vi "TAS-multiwavelength.vi"() -> ()   [LabVIEW 2012]
uses:
  <vilib>/DAQmx/read.llb/DAQmx Read (Analog DBL 1Chan 1Samp).vi
  <vilib>/DAQmx/miscellaneous.llb/DAQmx Fill In Error Info.vi
panel:
  out "Light Level":cluster{"X":dbl, "Y":dbl}[](graph)
  in  "ABORT LL SCAN":bool
  out "Monos moving":bool
  out "error out 2":errorcluster
  out "error out":errorcluster
  out "Detector Blaze":dbl
  out "Lamp Blaze":dbl
  out "Lamp WL":dbl
  out "Detector WL":dbl
  out "Laser Shutter State":string
  in  "START SCAN":bool
  out "Scanning":bool
  out "Osc. Time Range":string
  out "Laser State":string
  out "Total Steps":string
  out "Current Step":string
  out "Light Level (V)":dbl
  out "OPO Shutter State":string
  out "Total Averages":string
  out "Current Average":string
  out "Detector State":string
  out "Lamp State":string
  in  "SetTimeRange":bool
  in  "Time range":string(combo)
  in  "Averages per WL":dbl
  in  "Change Grating":bool
  in  "ScanLightLevel":bool
  in  "SAVE":bool
  in  "LASER OFF":bool
  in  "ABORT SCAN":bool
  in  "LASER ON":bool
  in  "Grating choice":dbl=1.0 min=1.0 max=2.0 step=1.0
  in  "Wavelength Range":string
  out "Scan Progress":u8(slide) scale=0.0..100.0
  in  "Exit":bool
  out "Transient Absorption":dbl[][](graph)
  # "Current state"
  # "WARNING: THIS PROGRAM IS UNDER\nDEVELOPMENT AND MUST NOT BE USED"
  # "Wavelength Settings"
  # "MATLAB notation. Leave a gap\nat the excitation WL. Example:\n\"300:1:450 500:1:700\" scans 300-450nm with a step of 1nm, leaves\na 50 nm gap around the excitation WL 475 nm, then continues scanning 500-700nm with a step of 1 nm."
  # "Maximum transmission occurs at\nblaze WL.\n\nBlaze 1 = 350 nm, Blaze 2 = 750 nm."
  # "Time range and averaging"
  # "Reserved For Future Convenience Functions"
  # "System"
  # "Light Level"
  # "Check if the light level is good over the\nselected wavelength range. Optimum 1.25 V, don't exceed 1.5 V at any WL."
  # "Remember to set the filter knobs manually according to table:"
  # "Time Range:          High Pass:          Low Pass:\n100 ns/div              10 us                   10 ns\n1 us/div                  100 us                 100 ns\n10 us/div                1 ms                    1 us\n100 us/div              10 ms                  10 us"
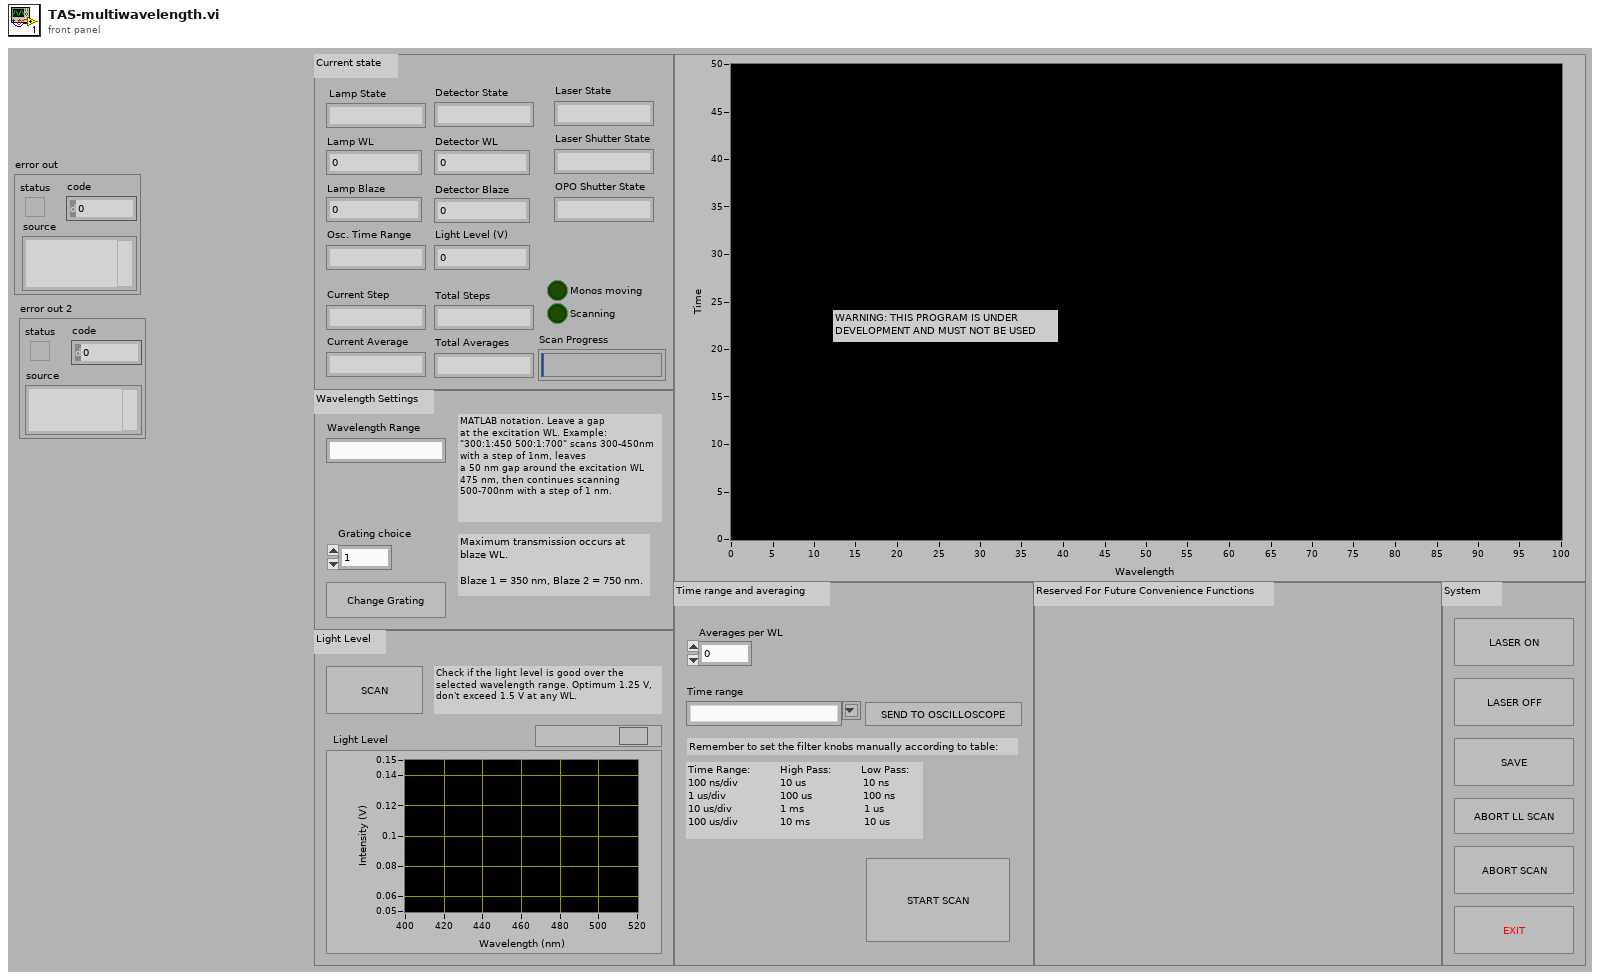
[diagram p1: front panel]
types:
  T1 = typedef "Cornerstone deviceID.ctl" = i32
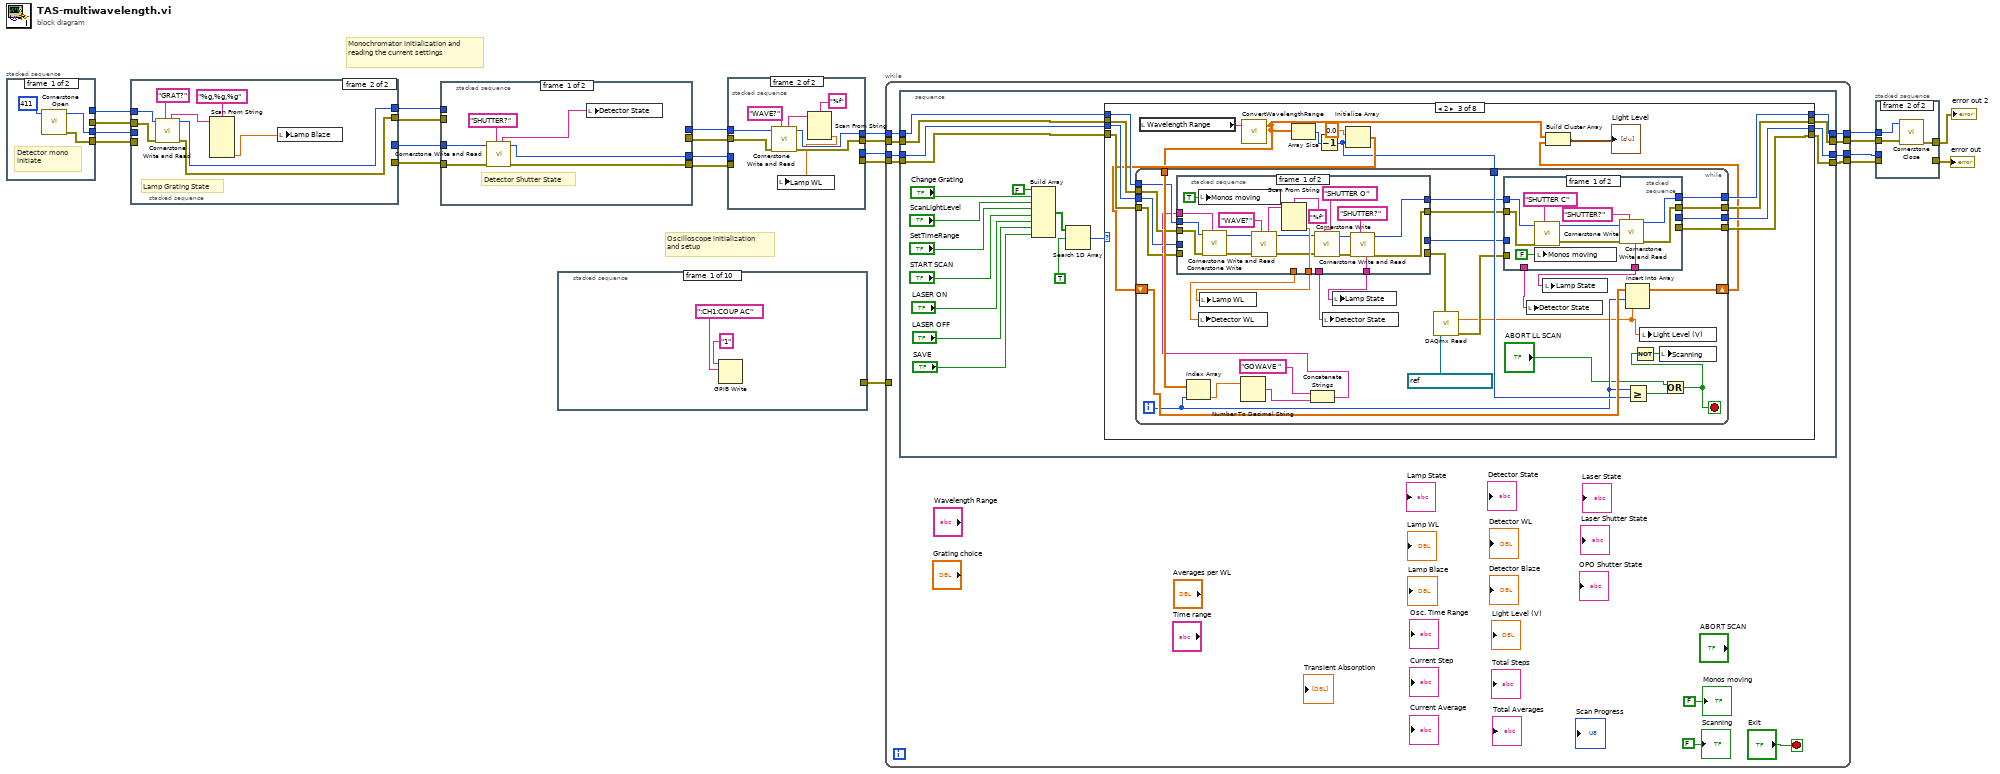
[diagram p0: block diagram]
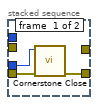
[diagram p2: hidden frame]
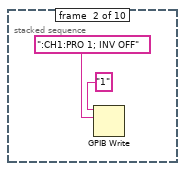
[diagram p3: hidden frame]
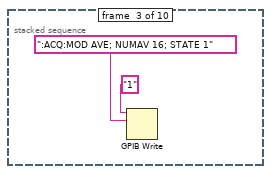
[diagram p4: hidden frame]
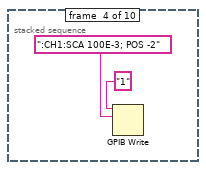
[diagram p5: hidden frame]
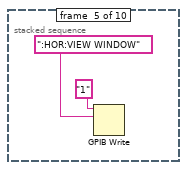
[diagram p6: hidden frame]
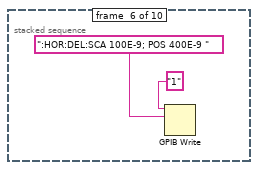
[diagram p7: hidden frame]
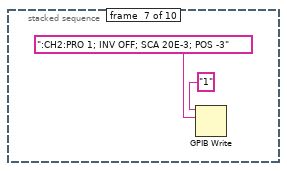
[diagram p8: hidden frame]
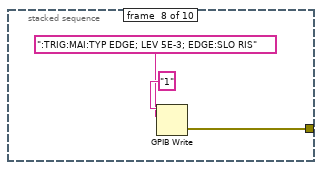
[diagram p9: hidden frame]
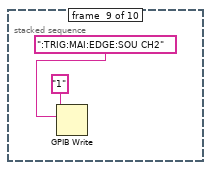
[diagram p10: hidden frame]
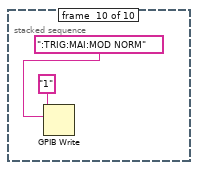
[diagram p11: hidden frame]
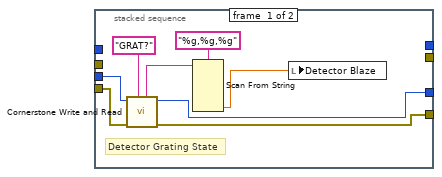
[diagram p12: hidden frame]
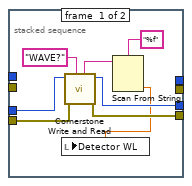
[diagram p13: hidden frame]
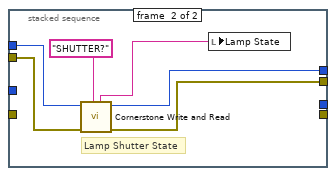
[diagram p14: hidden frame]
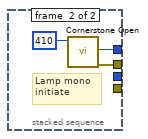
[diagram p15: hidden frame]
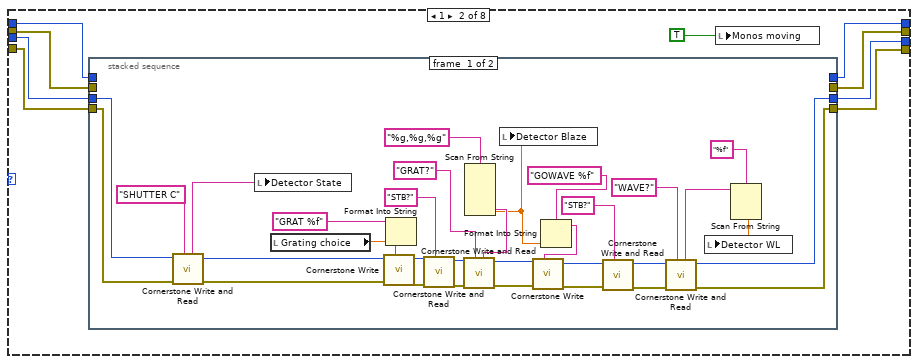
[diagram p17: hidden frame]
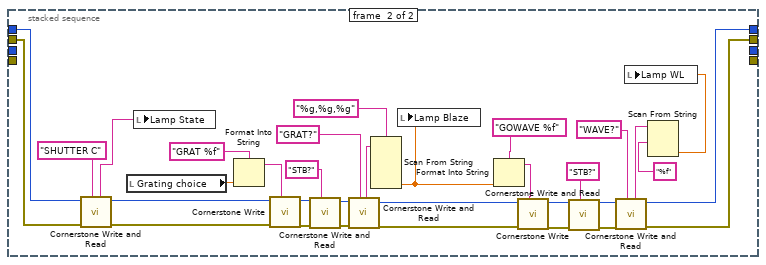
[diagram p18: hidden frame]
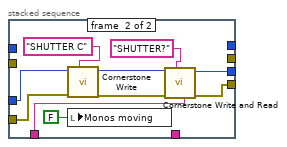
[diagram p19: hidden frame]
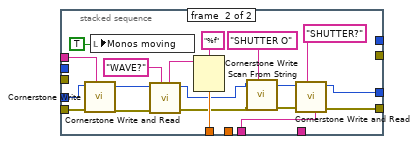
[diagram p20: hidden frame]
diagram:
  # "Oscilloscope initialization\nand setup"
  # "Monochromator initialization and reading the current settings"
  n1 = stacked-sequence {
    tunnel: [_ w28] -> w16
    tunnel: [_ w27] -> w17
    tunnel: [w25 _] -> w22
    tunnel: [w24 _] -> w23
    frame #0 {
      # "Detector mono\ninitiate"
      n2 = call "Cornerstone Open.vi"("serial # (0: first device)"=u32 411 ("serial #")) -> ("error out"=w24:errorcluster, "cs_deviceID"=w25:T1)  [unwired: 9 in]
    }
    frame #1 {
      # "Lamp mono\ninitiate"
      n3 = call "Cornerstone Open.vi"("serial # (0: first device)"=u32 410 ("serial #")) -> ("error out"=w28:errorcluster, "cs_deviceID"=w27:T1)  [unwired: 9 in]
    }
  }
  n4 = stacked-sequence {
    tunnel: [_ w42] -> w15
    tunnel: [_ w41] -> w14
    tunnel: w17 -> [_ w40]
    tunnel: w16 -> [_ w39]
    tunnel: w22 -> [w34 _]
    tunnel: w23 -> [w33 _]
    tunnel: [w32 _] -> w21
    tunnel: [w31 _] -> w20
    frame #0 {
      # "Detector Grating State"
      n5 = call "Cornerstone Write and Read.vi"("statement"="GRAT?", "error in (no error)"=w33, "cs_deviceID"=w34) -> ("error out"=w32:errorcluster, "passed cs_deviceID"=w31:T1, "response"=w36:string)  [unwired: 4 in]
      n6 = Scan From String(format string="%g,%g,%g", input string=w36) -> (output 3=w30:dbl)  [unwired: 7 in, 3 out]
      n7 = local write "Detector Blaze"(w30) -> ()
    }
    frame #1 {
      # "Lamp Grating State"
      n8 = call "Cornerstone Write and Read.vi"("statement"="GRAT?", "error in (no error)"=w39, "cs_deviceID"=w40) -> ("error out"=w41:errorcluster, "passed cs_deviceID"=w42:T1, "response"=w44:string)  [unwired: 4 in]
      n9 = Scan From String(format string="%g,%g,%g", input string=w44) -> (output 3=w38:dbl)  [unwired: 7 in, 3 out]
      n10 = local write "Lamp Blaze"(w38) -> ()
    }
  }
  n11 = stacked-sequence {
    tunnel: w20 -> [w50 _]
    tunnel: w21 -> [w49 _]
    tunnel: w15 -> [_ w56]
    tunnel: w14 -> [_ w55]
    tunnel: [w48 _] -> w19
    tunnel: [w47 _] -> w18
    tunnel: [_ w54] -> w12
    tunnel: [_ w53] -> w13
    frame #0 {
      # "Detector Shutter State"
      n12 = call "Cornerstone Write and Read.vi"("statement"="SHUTTER?", "error in (no error)"=w49, "cs_deviceID"=w50) -> ("error out"=w48:errorcluster, "passed cs_deviceID"=w47:T1, "response"=w46:string)  [unwired: 4 in]
      n13 = local write "Detector State"(w46) -> ()
    }
    frame #1 {
      # "Lamp Shutter State"
      n14 = call "Cornerstone Write and Read.vi"("statement"="SHUTTER?", "error in (no error)"=w55, "cs_deviceID"=w56) -> ("error out"=w53:errorcluster, "passed cs_deviceID"=w54:T1, "response"=w52:string)  [unwired: 4 in]
      n15 = local write "Lamp State"(w52) -> ()
    }
  }
  n16 = stacked-sequence {
    tunnel: [_ _ _ _ _ _ _ w72 _ _] -> w1
    frame #0 {
      n17 = GPIB Write(0:"1" ("address string"), 1:":CH1:COUP AC" ("data")) -> ()  [unwired: 3 in, 2 out]
    }
    frame #1 {
      n18 = GPIB Write(0:"1" ("address string"), 1:":CH1:PRO 1; INV OFF" ("data")) -> ()  [unwired: 3 in, 2 out]
    }
    frame #2 {
      n19 = GPIB Write(0:"1" ("address string"), 1:":ACQ:MOD AVE; NUMAV 16; STATE 1" ("data")) -> ()  [unwired: 3 in, 2 out]
    }
    frame #3 {
      n20 = GPIB Write(0:"1" ("address string"), 1:":CH1:SCA 100E-3; POS -2" ("data")) -> ()  [unwired: 3 in, 2 out]
    }
    frame #4 {
      n21 = GPIB Write(0:"1" ("address string"), 1:":HOR:VIEW WINDOW" ("data")) -> ()  [unwired: 3 in, 2 out]
    }
    frame #5 {
      n22 = GPIB Write(0:"1" ("address string"), 1:":HOR:DEL:SCA 100E-9; POS 400E-9 " ("data")) -> ()  [unwired: 3 in, 2 out]
    }
    frame #6 {
      n23 = GPIB Write(0:"1" ("address string"), 1:":CH2:PRO 1; INV OFF; SCA 20E-3; POS -3" ("data")) -> ()  [unwired: 3 in, 2 out]
    }
    frame #7 {
      n24 = GPIB Write(0:"1" ("address string"), 1:":TRIG:MAI:TYP EDGE; LEV 5E-3; EDGE:SLO RIS" ("data")) -> (6:w72:errorcluster)  [unwired: 3 in, 1 out]
    }
    frame #8 {
      n25 = GPIB Write(0:"1" ("address string"), 1:":TRIG:MAI:EDGE:SOU CH2" ("data")) -> ()  [unwired: 3 in, 2 out]
    }
    frame #9 {
      n26 = GPIB Write(0:"1" ("address string"), 1:":TRIG:MAI:MOD NORM" ("data")) -> ()  [unwired: 3 in, 2 out]
    }
  }
  n27 = stacked-sequence {
    tunnel: w19 -> [w83 _]
    tunnel: w18 -> [w82 _]
    tunnel: [w81 _] -> w9
    tunnel: [w80 _] -> w4
    tunnel: w12 -> [_ w91]
    tunnel: w13 -> [_ w90]
    tunnel: [_ w89] -> w3
    tunnel: [_ w88] -> w7
    frame #0 {
      n28 = call "Cornerstone Write and Read.vi"("statement"="WAVE?", "error in (no error)"=w83, "cs_deviceID"=w82) -> ("error out"=w81:errorcluster, "passed cs_deviceID"=w80:T1, "response"=w84:string)  [unwired: 4 in]
      n29 = Scan From String(format string="%f", input string=w84) -> (output 1=w79:dbl)  [unwired: 3 in, 3 out]
      n30 = local write "Detector WL"(w79) -> ()
    }
    frame #1 {
      n31 = call "Cornerstone Write and Read.vi"("statement"="WAVE?", "error in (no error)"=w90, "cs_deviceID"=w91) -> ("error out"=w88:errorcluster, "passed cs_deviceID"=w89:T1, "response"=w94:string)  [unwired: 4 in]
      n32 = Scan From String(format string="%f", input string=w94) -> (output 1=w87:dbl)  [unwired: 3 in, 3 out]
      n33 = local write "Lamp WL"(w87) -> ()
    }
  }
  n34 = while {
    tunnel: [w96] -> w8
    tunnel: w9 -> [w98]
    tunnel: [w100] -> w6
    tunnel: w7 -> [w101]
    tunnel: w4 -> [w99]
    tunnel: [w97] -> w5
    tunnel: [w102] -> w2
    tunnel: w3 -> [w103]
    tunnel: w1 -> [_]
    stop <- "Exit" stop-if-true
    n35 = stacked-sequence {
      tunnel: w103 -> [w124]
      tunnel: [w121] -> w102
      tunnel: w101 -> [w123]
      tunnel: [w120] -> w100
      tunnel: w99 -> [w106]
      tunnel: w98 -> [w122]
      tunnel: [w119] -> w97
      tunnel: [w118] -> w96
      frame #0 {
        n36 = Build Array(FALSE ("element"), "Change Grating", "ScanLightLevel", "SetTimeRange", "START SCAN", "LASER ON", "LASER OFF", "SAVE") -> (w117:bool[])
        n37 = Search 1D Array(1D array=w117, element=TRUE) -> (index of element=w116:i32)  [unwired: 1 in]
        n38 = case shown="2" w116 {
          tunnel: w124 -> [w128 w136 w215 w321 w325 w332 w339 w340]
          tunnel: w123 -> [w127 w133 w216 w320 w324 w331 w338 w343]
          tunnel: w106 -> [w126 w131 w217 w319 w323 w330 w337 w342]
          tunnel: w122 -> [w125 w130 w218 w314 w322 w329 w336 w341]
          tunnel: [w128 w135 w212 w321 w325 w332 w339 w340] -> w121
          tunnel: [w127 w134 w211 w320 w324 w331 w338 w343] -> w120
          tunnel: [w126 w132 w210 w319 w323 w330 w337 w342] -> w119
          tunnel: [w125 w129 w209 w317 w322 w329 w336 w341] -> w118
          frame 0, Default {
          }
          frame 1 {
            n39 = stacked-sequence {
              tunnel: w136 -> [_ w174]
              tunnel: [_ w187] -> w135
              tunnel: [_ w186] -> w134
              tunnel: w133 -> [_ w173]
              tunnel: [w145 _] -> w132
              tunnel: w131 -> [w141 _]
              tunnel: [w144 _] -> w129
              tunnel: w130 -> [w140 _]
              frame #0 {
                n40 = call "Cornerstone Write and Read.vi"("statement"="SHUTTER C", "error in (no error)"=w140, "cs_deviceID"=w141) -> ("error out"=w142:errorcluster, "passed cs_deviceID"=w143:T1, "response"=w138:string)  [unwired: 4 in]
                n41 = local write "Detector State"(w138) -> ()
                n42 = local read "Grating choice"() -> (w161:dbl)
                n43 = Format Into String(format string="GRAT %f", w161) -> (resulting string=w162:string)  [unwired: 2 in, 1 out]
                n44 = call "Cornerstone Write.vi"("statement"=w162, "error in (no error)"=w142, "cs_deviceID"=w143) -> ("error out"=w168:errorcluster, "passed cs_deviceID"=w169:T1)  [unwired: 5 in]
                n45 = call "Cornerstone Write and Read.vi"("statement"="STB?", "error in (no error)"=w168, "cs_deviceID"=w169) -> ("error out"=w167:errorcluster, "passed cs_deviceID"=w166:T1)  [unwired: 4 in, 1 out]
                n46 = call "Cornerstone Write and Read.vi"("statement"="GRAT?", "error in (no error)"=w167, "cs_deviceID"=w166) -> ("error out"=w155:errorcluster, "passed cs_deviceID"=w156:T1, "response"=w165:string)  [unwired: 4 in]
                n47 = Scan From String(format string="%g,%g,%g", input string=w165) -> (output 3=w159:dbl)  [unwired: 7 in, 3 out]
                n48 = local write "Detector Blaze"(w159) -> ()
                n49 = Format Into String(format string="GOWAVE %f", w159) -> (resulting string=w157:string)  [unwired: 2 in, 1 out]
                n50 = call "Cornerstone Write.vi"("statement"=w157, "error in (no error)"=w155, "cs_deviceID"=w156) -> ("error out"=w153:errorcluster, "passed cs_deviceID"=w154:T1)  [unwired: 5 in]
                n51 = call "Cornerstone Write and Read.vi"("statement"="STB?", "error in (no error)"=w153, "cs_deviceID"=w154) -> ("error out"=w150:errorcluster, "passed cs_deviceID"=w151:T1)  [unwired: 4 in, 1 out]
                n52 = call "Cornerstone Write and Read.vi"("statement"="WAVE?", "error in (no error)"=w150, "cs_deviceID"=w151) -> ("error out"=w144:errorcluster, "passed cs_deviceID"=w145:T1, "response"=w148:string)  [unwired: 4 in]
                n53 = Scan From String(format string="%f", input string=w148) -> (output 1=w146:dbl)  [unwired: 3 in, 3 out]
                n54 = local write "Detector WL"(w146) -> ()
              }
              frame #1 {
                n55 = call "Cornerstone Write and Read.vi"("statement"="SHUTTER C", "error in (no error)"=w173, "cs_deviceID"=w174) -> ("error out"=w175:errorcluster, "passed cs_deviceID"=w176:T1, "response"=w171:string)  [unwired: 4 in]
                n56 = local read "Grating choice"() -> (w193:dbl)
                n57 = local write "Lamp State"(w171) -> ()
                n58 = Format Into String(format string="GRAT %f", w193) -> (resulting string=w202:string)  [unwired: 2 in, 1 out]
                n59 = call "Cornerstone Write.vi"("statement"=w202, "error in (no error)"=w175, "cs_deviceID"=w176) -> ("error out"=w196:errorcluster, "passed cs_deviceID"=w195:T1)  [unwired: 5 in]
                n60 = call "Cornerstone Write and Read.vi"("statement"="STB?", "error in (no error)"=w196, "cs_deviceID"=w195) -> ("error out"=w197:errorcluster, "passed cs_deviceID"=w198:T1)  [unwired: 4 in, 1 out]
                n61 = call "Cornerstone Write and Read.vi"("statement"="GRAT?", "error in (no error)"=w197, "cs_deviceID"=w198) -> ("error out"=w180:errorcluster, "passed cs_deviceID"=w181:T1, "response"=w199:string)  [unwired: 4 in]
                n62 = Scan From String(format string="%g,%g,%g", input string=w199) -> (output 3=w178:dbl)  [unwired: 7 in, 3 out]
                n63 = local write "Lamp Blaze"(w178) -> ()
                n64 = Format Into String(format string="GOWAVE %f", w178) -> (resulting string=w177:string)  [unwired: 2 in, 1 out]
                n65 = call "Cornerstone Write.vi"("statement"=w177, "error in (no error)"=w180, "cs_deviceID"=w181) -> ("error out"=w183:errorcluster, "passed cs_deviceID"=w182:T1)  [unwired: 5 in]
                n66 = call "Cornerstone Write and Read.vi"("statement"="STB?", "error in (no error)"=w183, "cs_deviceID"=w182) -> ("error out"=w184:errorcluster, "passed cs_deviceID"=w185:T1)  [unwired: 4 in, 1 out]
                n67 = call "Cornerstone Write and Read.vi"("statement"="WAVE?", "error in (no error)"=w184, "cs_deviceID"=w185) -> ("error out"=w186:errorcluster, "passed cs_deviceID"=w187:T1, "response"=w189:string)  [unwired: 4 in]
                n68 = Scan From String(format string="%f", input string=w189) -> (output 1=w179:dbl)  [unwired: 3 in, 3 out]
                n69 = local write "Lamp WL"(w179) -> ()
              }
            }
            n70 = local write "Monos moving"(TRUE ("Monos moving")) -> ()
          }
          frame 2 {
            n71 = local read "Wavelength Range"() -> (w219:string)
            n72 = call "ConvertWavelengthRange.vi"("UserString"=w219) -> ("Array"=w206:dbl[])  [unwired: 1 in, 1 out]
            n73 = Array Size(array=w206) -> (size(s)=w207:i32)
            n74 = Decrement(x=w207) -> (x-1=w208:i32)
            n75 = Initialize Array(0.0 ("element"), w208) -> (w213:dbl[])
            n76 = while {
              tunnel: w218 -> [w248]
              tunnel: w217 -> [w249]
              tunnel: w216 -> [w250]
              tunnel: w215 -> [w251]
              tunnel: w206 -> [w252]
              shift-right: [w246] -> w205
              shift-left: w213 -> [w247]
              tunnel: w208 -> [w245]
              tunnel: [w239] -> w212
              tunnel: [w238] -> w211
              tunnel: [w237] -> w210
              tunnel: [w236] -> w209
              i -> [w225]
              stop <- w223 stop-if-true
              n77 = Index Array(array=w252, index=w225) -> (element=w221:dbl)
              n78 = Number To Decimal String(number=w221) -> (decimal integer string=w232:string)  [unwired: 1 in]
              n79 = Concatenate Strings("GOWAVE " ("initial string"), w232) -> (w230:string)
              n80 = stacked-sequence {
                tunnel: w230 -> [w292 w311]
                tunnel: w251 -> [w291 _]
                tunnel: w250 -> [w290 _]
                tunnel: w249 -> [_ w310]
                tunnel: w248 -> [_ w309]
                tunnel: [w287 _] -> w244
                tunnel: [_ w303] -> w243
                tunnel: [_ w293] -> w233
                tunnel: [_ w294] -> w235
                tunnel: [w274 _] -> w241
                tunnel: [w275 _] -> w240
                tunnel: [w276 _] -> w229
                tunnel: [_ w296] -> w228
                frame #0 {
                  n81 = local write "Monos moving"(TRUE ("Monos moving")) -> ()
                  n82 = call "Cornerstone Write.vi"("statement"=w292, "error in (no error)"=w290, "cs_deviceID"=w291) -> ("error out"=w288:errorcluster, "passed cs_deviceID"=w289:T1)  [unwired: 5 in]
                  n83 = call "Cornerstone Write and Read.vi"("statement"="WAVE?", "error in (no error)"=w288, "cs_deviceID"=w289) -> ("error out"=w281:errorcluster, "passed cs_deviceID"=w282:T1, "response"=w286:string)  [unwired: 4 in]
                  n84 = Scan From String(format string="%f", input string=w286) -> (output 1=w287:dbl)  [unwired: 3 in, 3 out]
                  n85 = call "Cornerstone Write.vi"("statement"="SHUTTER O", "error in (no error)"=w281, "cs_deviceID"=w282) -> ("error out"=w278:errorcluster, "passed cs_deviceID"=w279:T1)  [unwired: 5 in]
                  n86 = call "Cornerstone Write and Read.vi"("statement"="SHUTTER?", "error in (no error)"=w278, "cs_deviceID"=w279) -> ("error out"=w274:errorcluster, "passed cs_deviceID"=w275:T1, "response"=w276:string)  [unwired: 4 in]
                }
                frame #1 {
                  n87 = call "Cornerstone Write.vi"("statement"=w311, "error in (no error)"=w309, "cs_deviceID"=w310) -> ("error out"=w307:errorcluster, "passed cs_deviceID"=w308:T1)  [unwired: 5 in]
                  n88 = local write "Monos moving"(TRUE ("Monos moving")) -> ()
                  n89 = call "Cornerstone Write and Read.vi"("statement"="WAVE?", "error in (no error)"=w307, "cs_deviceID"=w308) -> ("error out"=w300:errorcluster, "passed cs_deviceID"=w301:T1, "response"=w304:string)  [unwired: 4 in]
                  n90 = Scan From String(format string="%f", input string=w304) -> (output 1=w303:dbl)  [unwired: 3 in, 3 out]
                  n91 = call "Cornerstone Write.vi"("statement"="SHUTTER O", "error in (no error)"=w300, "cs_deviceID"=w301) -> ("error out"=w297:errorcluster, "passed cs_deviceID"=w298:T1)  [unwired: 5 in]
                  n92 = call "Cornerstone Write and Read.vi"("statement"="SHUTTER?", "error in (no error)"=w297, "cs_deviceID"=w298) -> ("error out"=w293:errorcluster, "passed cs_deviceID"=w294:T1, "response"=w296:string)  [unwired: 4 in]
                }
              }
              n93 = local write "Detector WL"(w243) -> ()
              n94 = local write "Lamp WL"(w244) -> ()
              n95 = local write "Detector State"(w228) -> ()
              n96 = local write "Lamp State"(w229) -> ()
              n97 = call-poly <vilib>:"DAQmx Read.vi"("task/channels in"=refnum<k21> "ai0_Light_Level", "error in"=w233) -> ("data"=w220:dbl, "error out"=w234:errorcluster)  [unwired: 11 in, 1 out]
              n98 = stacked-sequence {
                tunnel: w235 -> [_ w268]
                tunnel: w234 -> [_ w267]
                tunnel: w241 -> [w260 _]
                tunnel: w240 -> [w259 _]
                tunnel: [w263 _] -> w239
                tunnel: [w262 _] -> w238
                tunnel: [_ w273] -> w237
                tunnel: [_ w271] -> w236
                tunnel: [w254 _] -> w227
                tunnel: [_ w270] -> w226
                frame #0 {
                  n99 = call "Cornerstone Write.vi"("statement"="SHUTTER C", "error in (no error)"=w260, "cs_deviceID"=w259) -> ("error out"=w256:errorcluster, "passed cs_deviceID"=w257:T1)  [unwired: 5 in]
                  n100 = local write "Monos moving"(FALSE ("Monos moving")) -> ()
                  n101 = call "Cornerstone Write and Read.vi"("statement"="SHUTTER?", "error in (no error)"=w256, "cs_deviceID"=w257) -> ("error out"=w262:errorcluster, "passed cs_deviceID"=w263:T1, "response"=w254:string)  [unwired: 4 in]
                }
                frame #1 {
                  n102 = call "Cornerstone Write.vi"("statement"="SHUTTER C", "error in (no error)"=w267, "cs_deviceID"=w268) -> ("error out"=w265:errorcluster, "passed cs_deviceID"=w266:T1)  [unwired: 5 in]
                  n103 = local write "Monos moving"(FALSE ("Monos moving")) -> ()
                  n104 = call "Cornerstone Write and Read.vi"("statement"="SHUTTER?", "error in (no error)"=w265, "cs_deviceID"=w266) -> ("error out"=w271:errorcluster, "passed cs_deviceID"=w273:T1, "response"=w270:string)  [unwired: 4 in]
                }
              }
              n105 = local write "Detector State"(w226) -> ()
              n106 = local write "Lamp State"(w227) -> ()
              n107 = Insert Into Array(array=w247, index=w225, new element=w220) -> (w246:dbl[])
              n108 = Greater Or Equal?(x=w225, y=w245) -> (x >= y?=w224:bool)
              n109 = local write "Light Level (V)"(w220) -> ()
              n110 = Or(x="ABORT LL SCAN", y=w224) -> (x .or. y?=w223:bool)
              n111 = Not(x=w223) -> (.not. x?=w242:bool)
              n112 = local write "Scanning"(w242) -> ()
            }
            n113 = Build Cluster Array(w206, w205) -> (→"Light Level":cluster{"element":dbl, "element":dbl}[])
          }
          frame 3 {
            n114 = local read "Time range"() -> (w312:string)
            n115 = Format Into String(initial string="HORizontal:DELay:SCAle " ("data"), error in=w314, w312) -> (resulting string=w316:string, error out=w315:errorcluster)  [unwired: 1 in]
            n116 = GPIB Write(0:"1" ("address string"), 1:w316, 3:w315) -> (6:w317:errorcluster)  [unwired: 2 in, 1 out]
          }
          frame 4 {
          }
          frame 5 {
            # "Starts the laser"
            n117 = call "Serial Communication - Laser ML.vi"("Write String"="ST 1") -> ("error out"=w328:errorcluster)  [unwired: 1 in]
            n118 = call "Serial Communication - Laser ML.vi"("error in (no error)"=w328, "Write String"="ST 1") -> ()  [unwired: 1 out]
          }
          frame 6 {
            # "Turns the laser off"
            n119 = call "Serial Communication - Laser ML.vi"("Write String"="ST 0") -> ("error out"=w333:errorcluster)  [unwired: 1 in]
            n120 = call "Serial Communication - Laser ML.vi"("error in (no error)"=w333, "Write String"="ST 0") -> ()  [unwired: 1 out]
          }
          frame 7 {
          }
        }
      }
    }
    "Scanning" <- FALSE ("Scanning")
    "Monos moving" <- FALSE ("Monos moving")
  }
  n121 = stacked-sequence {
    tunnel: [w346 _] -> w11
    tunnel: w8 -> [w345 _]
    tunnel: w5 -> [w344 _]
    tunnel: w2 -> [_ w349]
    tunnel: w6 -> [_ w348]
    tunnel: [_ w347] -> w10
    frame #0 {
      n122 = call "Cornerstone Close.vi"("error in (ignored)"=w345, "cs_deviceID"=w344) -> ("error out"=w346:errorcluster)  [unwired: 9 in]
    }
    frame #1 {
      n123 = call "Cornerstone Close.vi"("error in (ignored)"=w348, "cs_deviceID"=w349) -> ("error out"=w347:errorcluster)  [unwired: 9 in]
    }
  }
  "error out" <- w11
  "error out 2" <- w10
